vi "PRL Configuration.vi"(8 "Error In":errorcluster, 11 "Configuration In":T1={"Connection Settings"={"IP-address"="127.0.0.1", "Port"="4711", "ID Code"=1001}, "Autostart"=FALSE, "Bad Data Removal"=TRUE, "Access Buffer Active"=TRUE, "Wait for Config Total Time [ms]"=2000, "Seconds to Wait if Config Fails [s]"=10, "Live Data Buffer Size"=5, "Number of Live Buffers in Access Buffer"=-1, "Data Rate History"=100, "Complex Data Points Allowed Equal"=10, "Analog Data Points Allowed Equal"=50, "Number of Connection Attempts"=3, "Access Queue Active"=FALSE, "Access Buffer Size [hh:mm]"=600.0, "Sampling rate [Hz]"=nan, "Manual Control"=FALSE, "dt Tolerance [microseconds]"=10.0, "Wait for Config Timeout [ms]"=20, "Max Time Stamp Age Before Reconnect [s]"=1.0, "Poll New Data Timeout [ms]"=5} {"Access Buffer Size [hh:mm]" format="%<%H:%M>t"}) -> (0 "Error Out":errorcluster, 3 "Configuration Out":T1={"Connection Settings"={"IP-address"="127.0.0.1", "Port"="4711", "ID Code"=1001}, "Autostart"=FALSE, "Bad Data Removal"=TRUE, "Access Buffer Active"=TRUE, "Wait for Config Total Time [ms]"=2000, "Seconds to Wait if Config Fails [s]"=10, "Live Data Buffer Size"=5, "Number of Live Buffers in Access Buffer"=-1, "Data Rate History"=100, "Complex Data Points Allowed Equal"=10, "Analog Data Points Allowed Equal"=50, "Number of Connection Attempts"=3, "Access Queue Active"=FALSE, "Access Buffer Size [hh:mm]"=600.0, "Sampling rate [Hz]"=50.0, "Manual Control"=FALSE, "dt Tolerance [microseconds]"=10.0, "Wait for Config Timeout [ms]"=20, "Max Time Stamp Age Before Reconnect [s]"=1.0, "Poll New Data Timeout [ms]"=5} {"Access Buffer Size [hh:mm]" format="%<%H:%M>t"})   [LabVIEW 2017, in "PMU Recorder Light.lvlib"]
uses:
  PMU Recorder Light.lvlib
panel:
  in  "Manual Control":bool
  in  "Cancel":bool
  in  "OK":bool
  in  "Tab":T2(tab)
  in  "Connection Settings":T3={"IP-address"="127.0.0.1", "Port"="8900", "ID Code"=1010}
  in  "Autostart":bool
  in  "Live Data Buffer Size\n[#data points]":i32=10
  in  "Access Buffer Active":bool=TRUE
  in  "Queue Active":bool=TRUE
  in  "Access Buffer Size\n[hh:mm:ss]":dbl=18000.0 format="%<%H:%M:%S>t"
  out "Data Points":i32=-1
  out "Buffer OK?":bool
  in  "dt Tolerance [microseconds]":dbl=10.0
  in  "Bad Data Removal":bool=TRUE
  in  "Analog Data Points Allowed Equal":i32=50
  in  "Complex Data Points Allowed Equal":i32=10
  in  "Poll New Data Timeout [ms]":u16=5
  in  "Max Time Stamp Age Before Reconnect [s]":dbl=5.0
  in  "Wait for Config Timeout [ms]":i32=2
  in  "Seconds to Try":dbl=2.0
  in  "Seconds to Wait Before Retry":dbl=10.0
  in  "Data Rate History":i32=100
  in  "DEPRECATED Number of Connection Attempts":i32=3
  in  "DEPRECATED Number of Live Buffers in Access Buffer":dbl=nan
  # "The live data buffer is used by both the queue and the\naccess buffer. It is filled by data directly from the \nC37.118 DLL. \nIt determines the number of data points to be read\nbefore the data is passed on. This will determine the\nmaximum update rate possible for the calling \nsoftware."
  # "Connection Details"
  # "Connection Details"
  # "Monitoring"
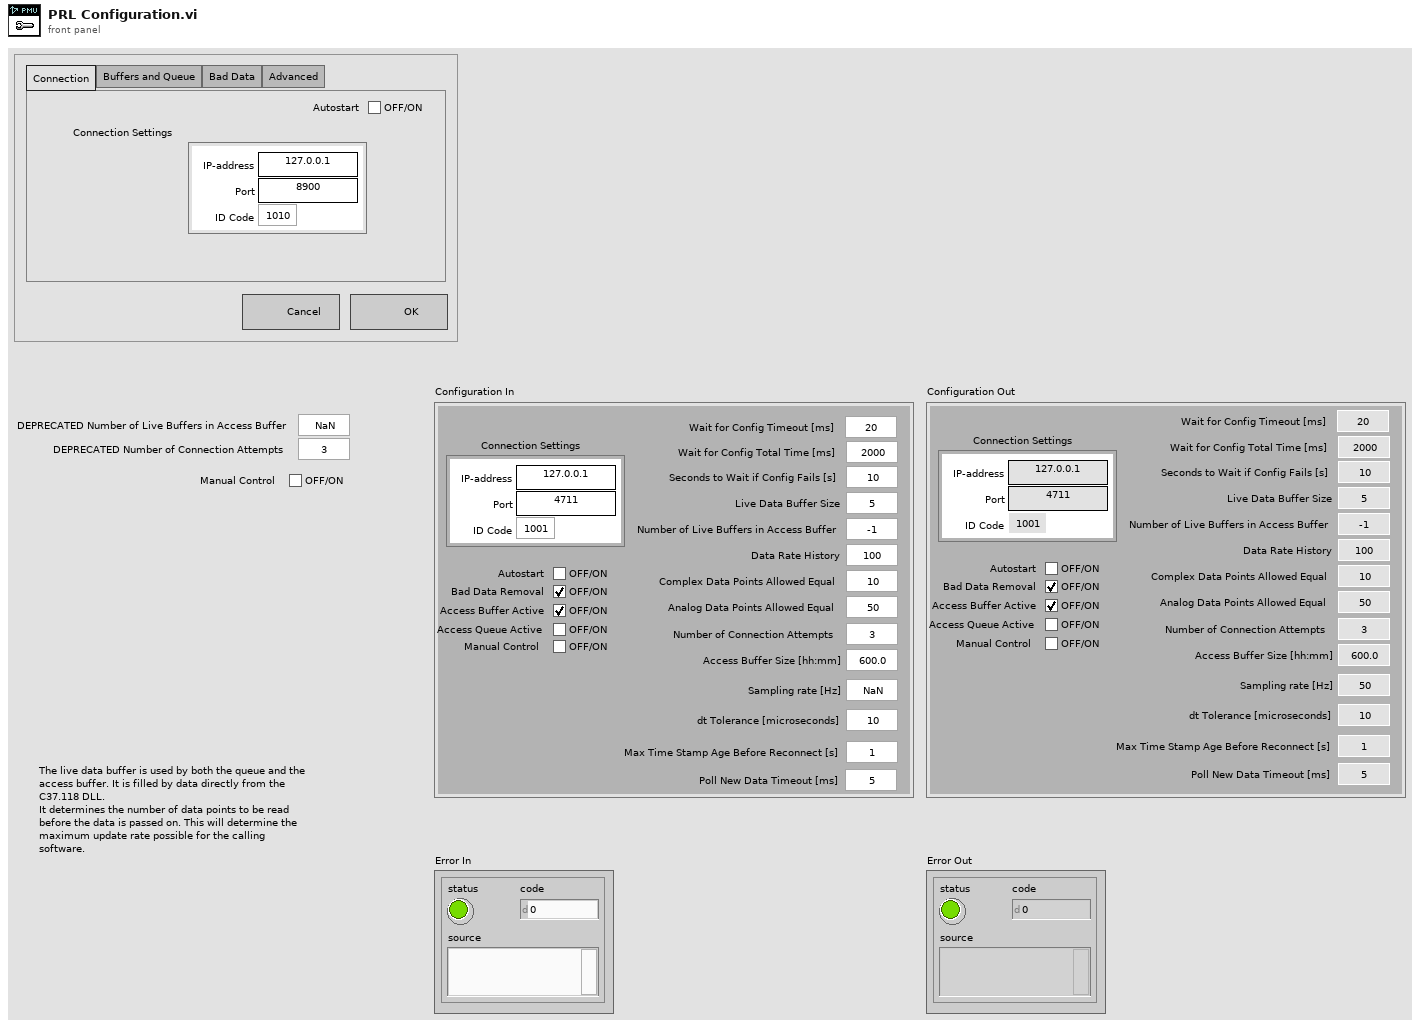
[diagram p1: front panel]
types:
  T1 = cluster{"Connection Settings":cluster{"IP-address":string, "Port":string, "ID Code":u32}, "Autostart":bool, "Bad Data Removal":bool, "Access Buffer Active":bool, "Wait for Config Total Time [ms]":i32, "Seconds to Wait if Config Fails [s]":i32, "Live Data Buffer Size":i32, "Number of Live Buffers in Access Buffer":i32, "Data Rate History":i32, "Complex Data Points Allowed Equal":i32, "Analog Data Points Allowed Equal":i32, "Number of Connection Attempts":i32, "Access Queue Active":bool, "Access Buffer Size [hh:mm]":dbl, "Sampling rate [Hz]":dbl, "Manual Control":bool, "dt Tolerance [microseconds]":dbl, "Wait for Config Timeout [ms]":i32, "Max Time Stamp Age Before Reconnect [s]":dbl, "Poll New Data Timeout [ms]":u16}
  T2 = enum32{"Connection", "Buffers and Queue", "Bad Data", "Advanced"}
  T3 = cluster{"IP-address":string, "Port":string, "ID Code":u32}
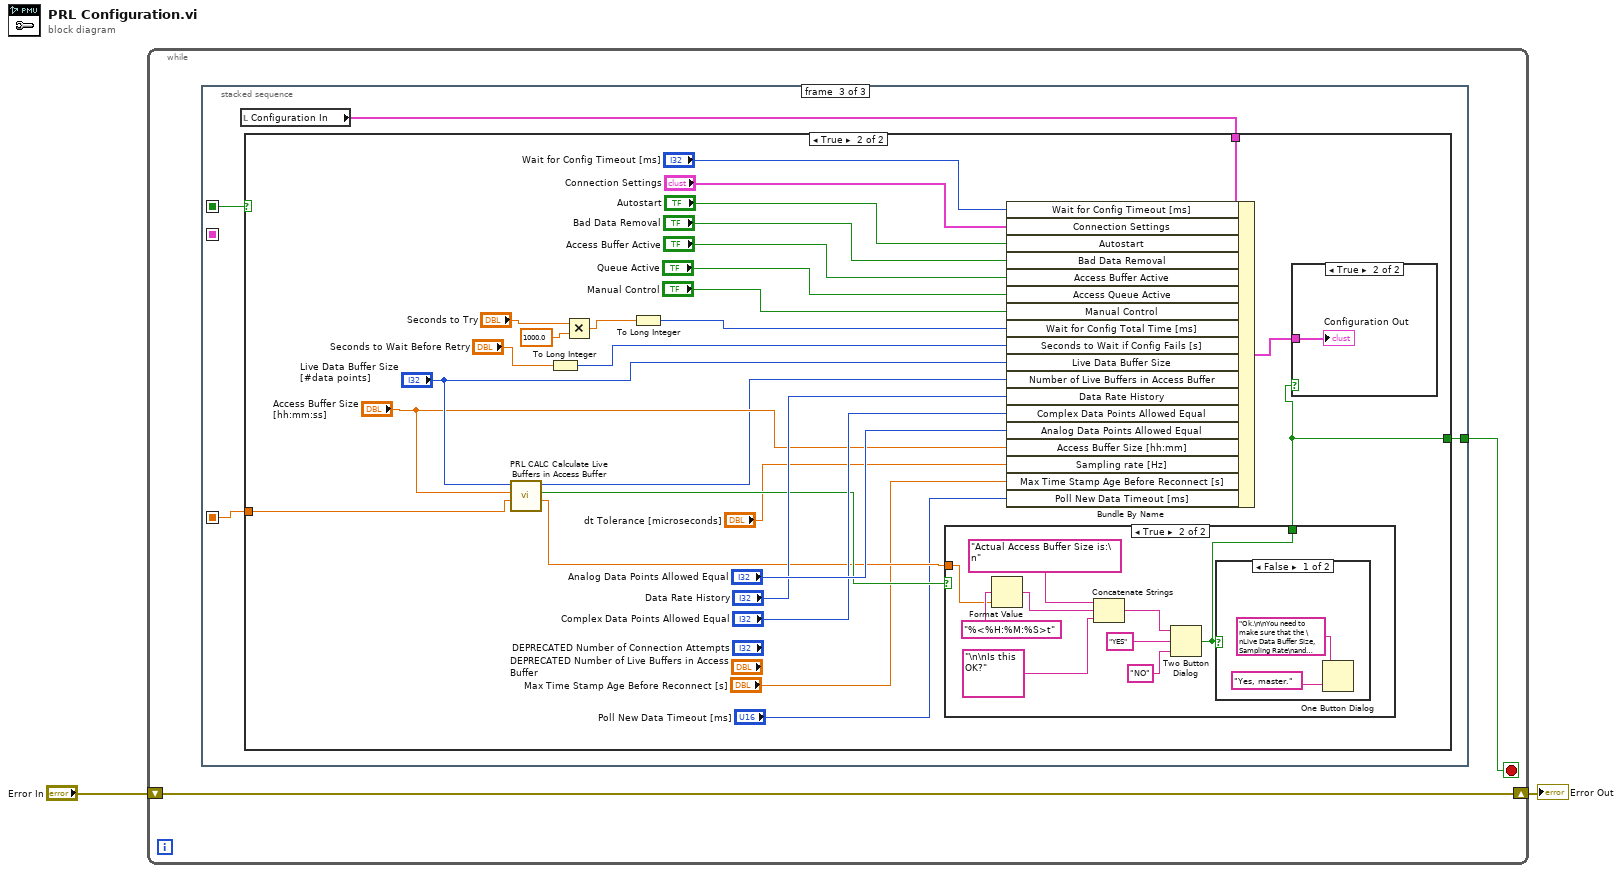
[diagram p0: block diagram]
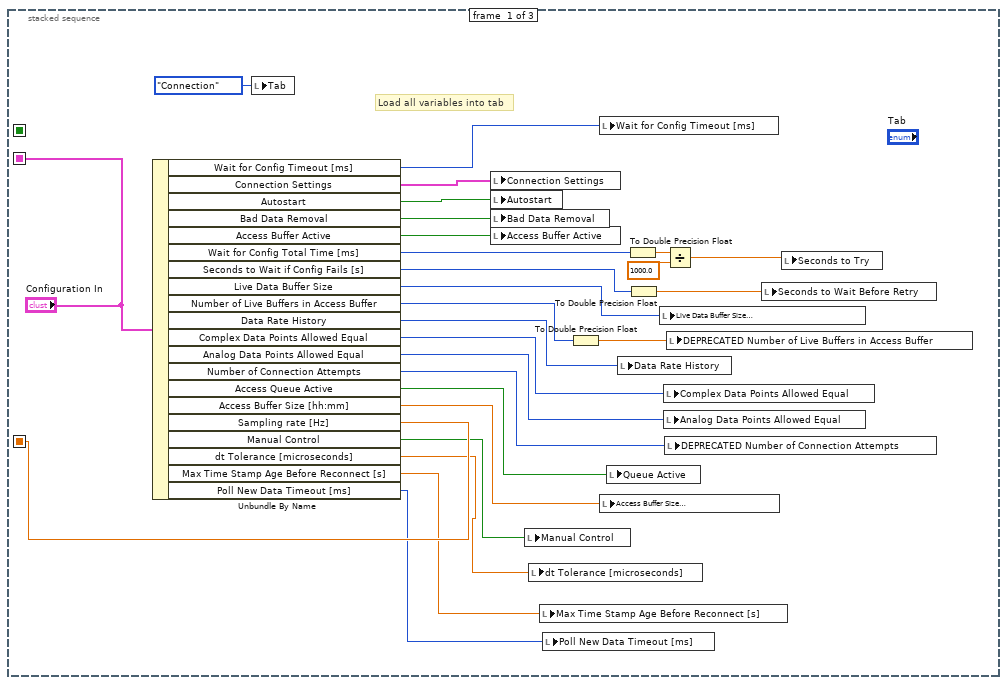
[diagram p2: hidden frame]
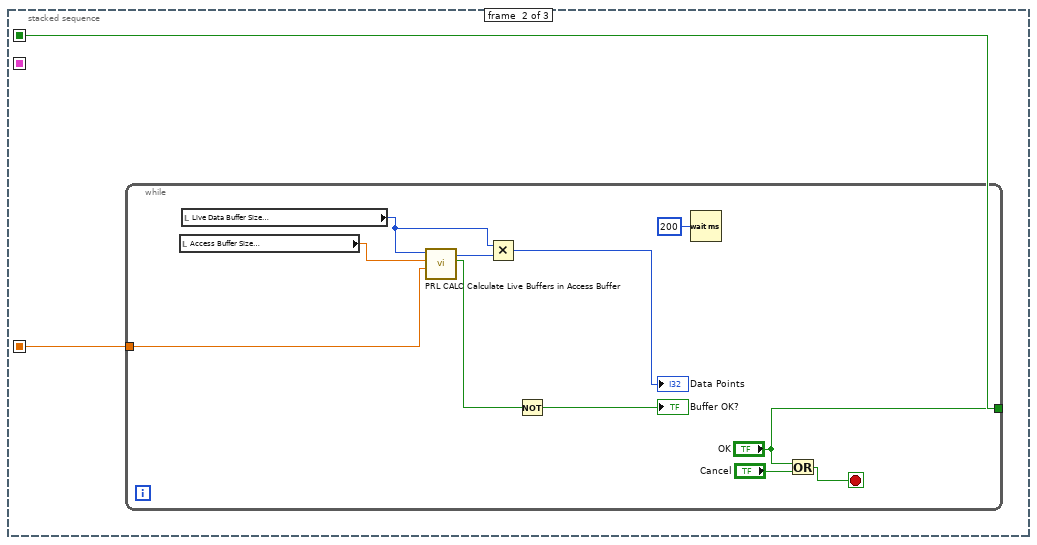
[diagram p3: hidden frame]
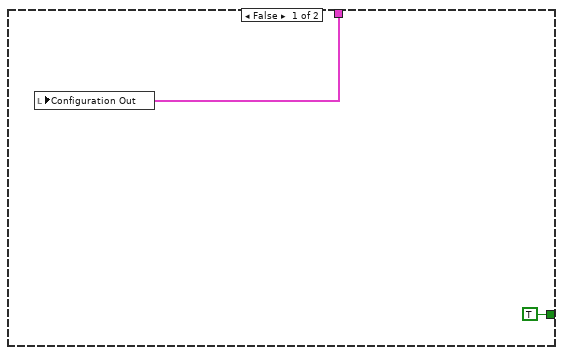
[diagram p4: hidden frame]
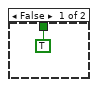
[diagram p6: hidden frame]
diagram:
  n1 = while {
    shift-right: [w3] -> w1
    shift-left: "Error In" -> [w3]
    stop <- w4 stop-if-true
    n2 = stacked-sequence {
      seq-local: [_ w33 _] -> [_ _ w48]
      seq-local: ["Configuration In" _ _] -> [_ _ _]
      seq-local: [w11 _ _] -> [_ w32 w47]
      tunnel: [_ _ w45] -> w4
      frame #0 {
        # "Load all variables into tab"
        n3 = Unbundle By Name("Configuration In") -> ("Wait for Config Timeout [ms]"=w7:i32, "Connection Settings"=w31:T3, "Autostart"=w30:bool, "Bad Data Removal"=w29:bool, "Access Buffer Active"=w28:bool, "Wait for Config Total Time [ms]"=w27:i32, "Seconds to Wait if Config Fails [s]"=w24:i32, "Live Data Buffer Size"=w15:i32, "Number of Live Buffers in Access Buffer"=w14:i32, "Data Rate History"=w20:i32, "Complex Data Points Allowed Equal"=w19:i32, "Analog Data Points Allowed Equal"=w18:i32, "Number of Connection Attempts"=w17:i32, "Access Queue Active"=w13:bool, "Access Buffer Size [hh:mm]"=w12:dbl, "Sampling rate [Hz]"=w11:dbl, "Manual Control"=w10:bool, "dt Tolerance [microseconds]"=w8:dbl, "Max Time Stamp Age Before Reconnect [s]"=w6:dbl, "Poll New Data Timeout [ms]"=w5:u16)
        n4 = local write "Tab"(T2."Connection" ("Tab")) -> ()
        n5 = local write "Connection Settings"(w31) -> ()
        n6 = local write "Autostart"(w30) -> ()
        n7 = local write "Bad Data Removal"(w29) -> ()
        n8 = local write "Access Buffer Active"(w28) -> ()
        n9 = local write "Manual Control"(w10) -> ()
        n10 = local write "dt Tolerance [microseconds]"(w8) -> ()
        n11 = local write "Max Time Stamp Age Before Reconnect [s]"(w6) -> ()
        n12 = local write "Poll New Data Timeout [ms]"(w5) -> ()
        n13 = To Double Precision Float(number=w14) -> (double precision float=w21:dbl)
        n14 = local write "Wait for Config Timeout [ms]"(w7) -> ()
        n15 = local write "Access Buffer Size\n[hh:mm:ss]"(w12) -> ()
        n16 = local write "Queue Active"(w13) -> ()
        n17 = local write "Data Rate History"(w20) -> ()
        n18 = To Double Precision Float(number=w27) -> (double precision float=w25:dbl)
        n19 = To Double Precision Float(number=w24) -> (double precision float=w22:dbl)
        n20 = local write "Live Data Buffer Size\n[#data points]"(w15) -> ()
        n21 = local write "Complex Data Points Allowed Equal"(w19) -> ()
        n22 = local write "Analog Data Points Allowed Equal"(w18) -> ()
        n23 = Divide(x=w25, y=1000.0) -> (x/y=w23:dbl)
        n24 = local write "DEPRECATED Number of Connection Attempts"(w17) -> ()
        n25 = local write "DEPRECATED Number of Live Buffers in Access Buffer"(w21) -> ()
        n26 = local write "Seconds to Wait Before Retry"(w22) -> ()
        n27 = local write "Seconds to Try"(w23) -> ()
      }
      frame #1 {
        n28 = while {
          tunnel: ["OK"] -> w33
          tunnel: w32 -> [w39]
          stop <- w43 stop-if-true
          n29 = local read "Access Buffer Size\n[hh:mm:ss]"() -> (w40:dbl)
          n30 = local read "Live Data Buffer Size\n[#data points]"() -> (w35:i32)
          n31 = call "PRL CALC Calculate Live Buffers in Access Buffer.vi"("Sampling rate [Hz]"=w39, "Access Buffer Size\n[hh:mm:ss]"=w40, "Live Data Buffer Size\n[#data points]"=w35) -> ("Buffer Mismatch"=w38:bool, "Number of Live Buffers in Access Buffer"=w36:i32)  [unwired: 6 in, 1 out]
          n32 = Multiply(x=w35, y=w36) -> (x*y=→"Data Points":i32)
          n33 = Not(x=w38) -> (.not. x?=→"Buffer OK?":bool)
          n34 = Wait (ms)(milliseconds to wait=u32 200) -> ()  [unwired: 1 out]
          n35 = Or(x="OK", y="Cancel") -> (x .or. y?=w43:bool)
        }
      }
      frame #2 {
        n36 = local read "Configuration In"() -> (w46:T1)
        n37 = case shown="True" w48 {
          tunnel: w46 -> [w49 w78]
          tunnel: w47 -> [_ w60]
          tunnel: [TRUE ("T button?") w63] -> w45
          frame False {
            n38 = local write "Configuration Out"(w49) -> ()
          }
          frame True {
            n39 = call "PRL CALC Calculate Live Buffers in Access Buffer.vi"("Sampling rate [Hz]"=w60, "Access Buffer Size\n[hh:mm:ss]"="Access Buffer Size\n[hh:mm:ss]", "Live Data Buffer Size\n[#data points]"="Live Data Buffer Size\n[#data points]") -> ("Actual Buffer Size"=w57:dbl, "Buffer Mismatch"=w59:bool, "Number of Live Buffers in Access Buffer"=w58:i32)  [unwired: 6 in]
            n40 = To Long Integer(number="Seconds to Wait Before Retry") -> (32bit integer=w68:i32)
            n41 = Multiply(x="Seconds to Try", y=1000.0) -> (x*y=w71:dbl)
            n42 = To Long Integer(number=w71) -> (32bit integer=w56:i32)
            n43 = case shown="True" w59 {
              tunnel: w57 -> [_ w88]
              tunnel: [TRUE ("T button?") w81] -> w63
              frame False {
              }
              frame True {
                n44 = Format Value(format string="%<%H:%M:%S>t", value (0)=w88) -> (output string=w86:string)  [unwired: 1 in]
                n45 = Concatenate Strings("Actual Access Buffer Size is:\n", w86, "\n\nIs this OK?") -> (w84:string)
                n46 = Two Button Dialog(message=w84, 1:"NO" ("F button name (\"Cancel\")"), 2:"YES" ("T button name (\"OK\")")) -> (T button?=w81:bool)
                n47 = case shown="False" w81 {
                  frame False {
                    n48 = One Button Dialog(message="Ok.\n\nYou need to make sure that the \nLive Data Buffer Size, Sampling Rate\nand Access Buffer Size allows for\nan integer number of data points\nin the buffer.\n", button name ("OK")="Yes, master.") -> ()  [unwired: 1 out]
                  }
                  frame True {
                  }
                }
              }
            }
            n49 = Bundle By Name(cluster=w78, "Wait for Config Timeout [ms]"="Wait for Config Timeout [ms]", "Connection Settings"="Connection Settings", "Autostart"="Autostart", "Bad Data Removal"="Bad Data Removal", "Access Buffer Active"="Access Buffer Active", "Access Queue Active"="Queue Active", "Manual Control"="Manual Control", "Wait for Config Total Time [ms]"=w56, "Seconds to Wait if Config Fails [s]"=w68, "Live Data Buffer Size"="Live Data Buffer Size\n[#data points]", "Number of Live Buffers in Access Buffer"=w58, "Data Rate History"="Data Rate History", "Complex Data Points Allowed Equal"="Complex Data Points Allowed Equal", "Analog Data Points Allowed Equal"="Analog Data Points Allowed Equal", "Access Buffer Size [hh:mm]"="Access Buffer Size\n[hh:mm:ss]", "Sampling rate [Hz]"="dt Tolerance [microseconds]", "Max Time Stamp Age Before Reconnect [s]"="Max Time Stamp Age Before Reconnect [s]", "Poll New Data Timeout [ms]"="Poll New Data Timeout [ms]") -> (w64:T1)
            n50 = case shown="True" w63 {
              tunnel: w64 -> [_ w79]
              frame False {
              }
              frame True {
                "Configuration Out" <- w79
              }
            }
          }
        }
      }
    }
  }
  "Error Out" <- w1
